vi "TEST Visualize File Merge.vi"() -> ()   [LabVIEW 2018, in "FileMerge.lvclass"]
uses:
  FileMerge.lvclass
panel:
  out "Num Sweeps 3":i32
  out "Num Sweeps 2":i32
  out "Num Sweeps":i32
  out "1 is sweeps are equal":i16[](graph)
  out "Merged File Timestamps":i32[](graph)
  out "Existing File Timestamps":i32[](graph)
  out "error out":errorcluster
  out "XY Graph":T1(graph)
  in  "Final, merged file path":path=path "C:/Users/Public/Documents/UCAR/APAR Board Test/DataFiles/2015-07-24_21_02_41MergeMaster4.csv"
  in  "ExistingFilePath":path=path "C:/Users/Public/Documents/UCAR/APAR Board Test/DataFiles/2015-07-24_21_02_41MergeMaster4.csv"
  # "Look at old file and  new file together."
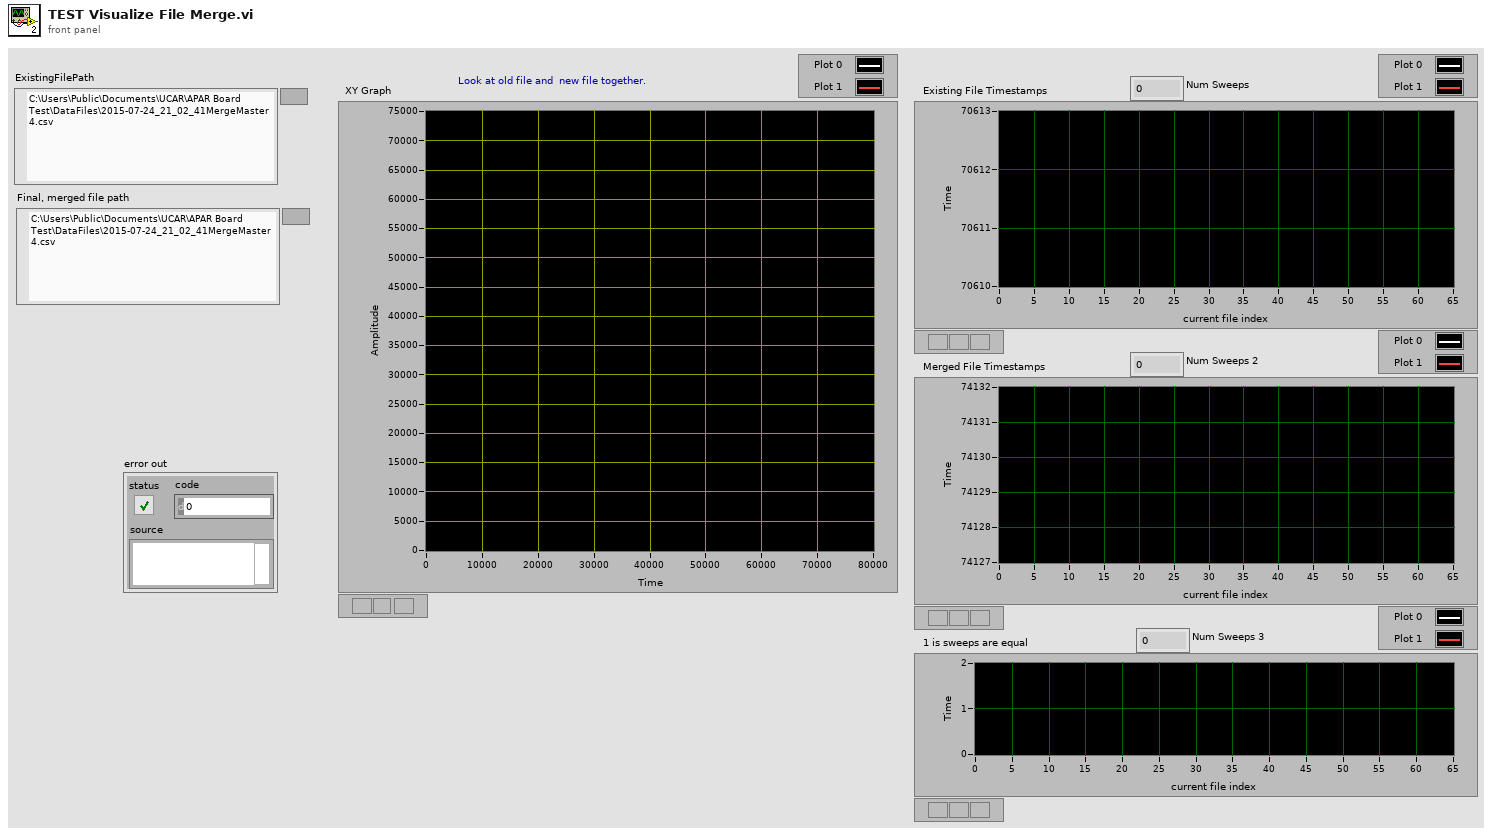
[diagram p1: front panel]
types:
  T1 = cluster{"Waveform Graph":i32[], "Waveform Graph":i32[]}[]
  T2 = cluster{"Sweep Number vs index in current file":i32[], "Sweep Number vs index in current file":i32[]}
  T3 = cluster{"Sweep Number vs index in current file":i32[], "Sweep Number vs index in current file":i32[]}[]
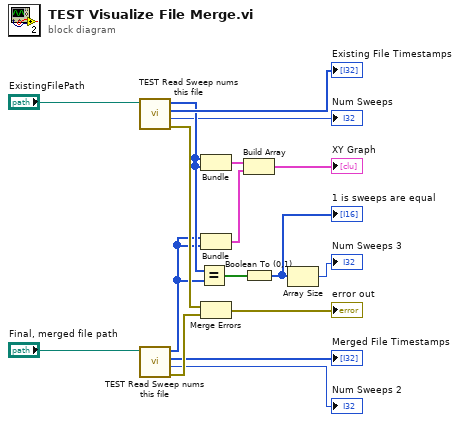
[diagram p0: block diagram]
diagram:
  n1 = call "TEST Read Sweep nums this file.vi"("ExistingFilePath"="ExistingFilePath") -> ("error out"=w12:errorcluster, "Num Sweeps"=→"Num Sweeps":i32, "Timestamp in s vs index in current file"=→"Existing File Timestamps":i32[], "Sweep Number vs index in current file"=w7:i32[])  [unwired: 6 in, 1 out]
  n2 = call "TEST Read Sweep nums this file.vi"("ExistingFilePath"="Final, merged file path") -> ("error out"=w11:errorcluster, "Num Sweeps"=→"Num Sweeps 2":i32, "Timestamp in s vs index in current file"=→"Merged File Timestamps":i32[], "Sweep Number vs index in current file"=w6:i32[])  [unwired: 6 in, 1 out]
  n3 = Equal?(x=w7, y=w6) -> (x = y?=w5:bool[])
  n4 = Bundle("Sweep Number vs index in current file"=w7, "Sweep Number vs index in current file"=w7) -> (w15:T2)  [unwired: 1 in]
  n5 = Bundle("Sweep Number vs index in current file"=w6, "Sweep Number vs index in current file"=w6) -> (w14:T2)  [unwired: 1 in]
  n6 = Merge Errors(w12, w11) -> (→"error out":errorcluster)
  n7 = Build Array(w15, w14) -> (→"XY Graph":T3)
  n8 = Boolean To (0,1)(Boolean=w5) -> (0, 1=w1:i16[])
  "1 is sweeps are equal" <- w1
  n9 = Array Size(array=w1) -> (size(s)=→"Num Sweeps 3":i32)
